vi "MKS CTLR - Check Channel Result.vi"(7 "Channel":T1(ring), 8 "error in (no error)":errorcluster, 11 "VISA resource name (IN)":refnum<visa-resource-name>) -> (0 "error out":errorcluster, 3 "VISA resource name (OUT)":refnum<visa-resource-name>, 4 "String Value":string, 5 "Pressure value":dbl)   [LabVIEW 2013]
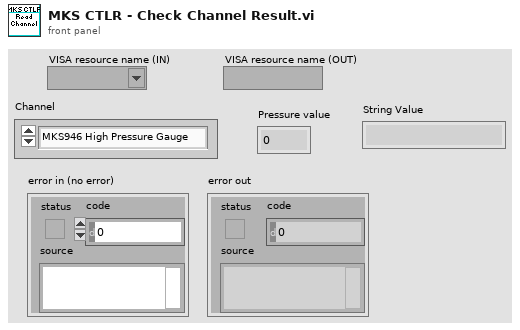
[diagram p1: front panel]
types:
  T1 = enum16{"MKS946 High Pressure Gauge", "MKS946 Separator Flow", "MKS946 Target Cavity Flow", "MKS670 Low Pressure Gauge"}
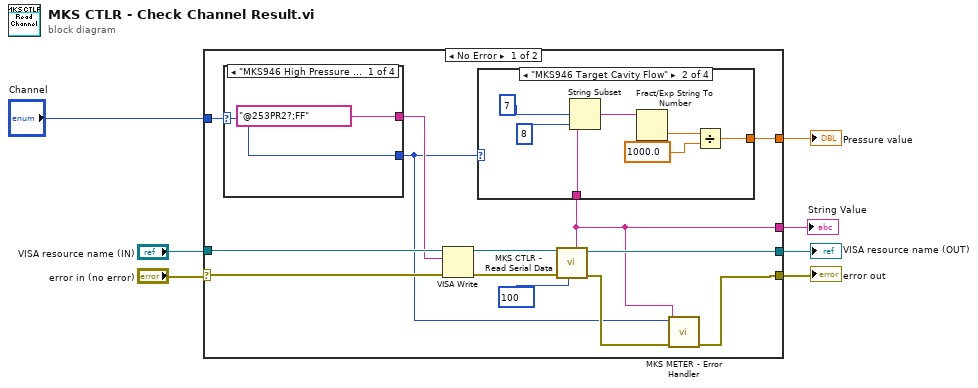
[diagram p0: block diagram]
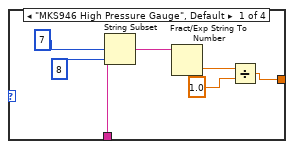
[diagram p2: hidden frame]
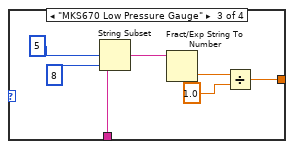
[diagram p3: hidden frame]
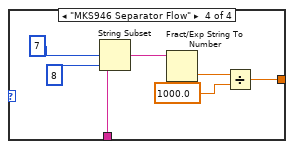
[diagram p4: hidden frame]
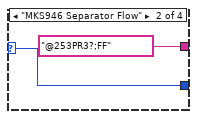
[diagram p5: hidden frame]
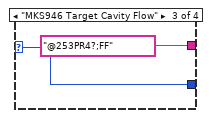
[diagram p6: hidden frame]
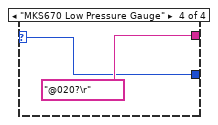
[diagram p7: hidden frame]
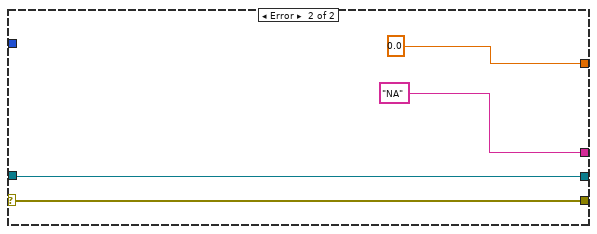
[diagram p8: hidden frame]
diagram:
  n1 = case shown="No Error" "error in (no error)" {
    selector: "error in (no error)" -> [w14 w60]
    tunnel: "VISA resource name (IN)" -> [w20 w59]
    tunnel: [w16 0.0] -> w6
    tunnel: [w10 w60] -> w5
    tunnel: [w15 w59] -> w4
    tunnel: [w9 "NA" ("Response")] -> w2
    tunnel: "Channel" -> [w12 _]
    frame No Error {
      n2 = case shown="\"MKS946 High Pressure Gauge\", Default" w12 {
        selector: w12 -> [w49 w51 w53 w55]
        tunnel: ["@253PR2?;FF" "@253PR3?;FF" "@253PR4?;FF" "@020?\r" ("Command")] -> w13
        tunnel: [w49 w51 w53 w55] -> w8
        frame "MKS946 High Pressure Gauge", Default {
        }
        frame "MKS946 Separator Flow" {
        }
        frame "MKS946 Target Cavity Flow" {
        }
        frame "MKS670 Low Pressure Gauge" {
        }
      }
      n3 = VISA Write(VISA resource name=w20, write buffer=w13, error in (no error)=w14) -> (VISA resource name out=w18:refnum<visa-resource-name>, error out=w19:errorcluster)  [unwired: 1 out]
      n4 = call "MKS CTLR - Read Serial Data.vi"("Read timeout (mSec)"=u64 100 ("Read timeout (Sec)"), "error in (no error)"=w19, "VISA resource name (IN)"=w18) -> ("error out"=w11:errorcluster, "VISA resource name (OUT)"=w15:refnum<visa-resource-name>, "Response"=w9:string)  [unwired: 6 in]
      n5 = case shown="\"MKS946 Target Cavity Flow\"" w8 {
        tunnel: [w22 w28 w35 w46] -> w16
        tunnel: w9 -> [w21 w29 w36 w44]
        frame "MKS946 High Pressure Gauge", Default {
          n6 = String Subset(string=w21, offset (0)=7 ("offset"), length (rest)=8 ("offset past number")) -> (substring=w25:string)
          n7 = Fract/Exp String To Number(string=w25) -> (number=w23:dbl)  [unwired: 3 in, 1 out]
          n8 = Divide(x=w23, y=1.0) -> (x/y=w22:dbl)
        }
        frame "MKS946 Target Cavity Flow" {
          n9 = String Subset(string=w29, offset (0)=7 ("offset"), length (rest)=8 ("offset past number")) -> (substring=w32:string)
          n10 = Fract/Exp String To Number(string=w32) -> (number=w30:dbl)  [unwired: 3 in, 1 out]
          n11 = Divide(x=w30, y=1000.0) -> (x/y=w28:dbl)
        }
        frame "MKS670 Low Pressure Gauge" {
          n12 = String Subset(string=w36, offset (0)=5 ("offset"), length (rest)=8 ("offset past number")) -> (substring=w39:string)
          n13 = Fract/Exp String To Number(string=w39) -> (number=w37:dbl)  [unwired: 3 in, 1 out]
          n14 = Divide(x=w37, y=1.0) -> (x/y=w35:dbl)
        }
        frame "MKS946 Separator Flow" {
          n15 = String Subset(string=w44, offset (0)=7 ("offset"), length (rest)=8 ("offset past number")) -> (substring=w45:string)
          n16 = Fract/Exp String To Number(string=w45) -> (number=w48:dbl)  [unwired: 3 in, 1 out]
          n17 = Divide(x=w48, y=1000.0) -> (x/y=w46:dbl)
        }
      }
      n18 = call "MKS METER - Error Handler.vi"("error in (no error)"=w11, "Channel String"=w9, "Channel"=w8) -> ("error out"=w10:errorcluster)  [unwired: 8 in]
    }
    frame Error {
    }
  }
  "error out" <- w5
  "VISA resource name (OUT)" <- w4
  "Pressure value" <- w6
  "String Value" <- w2
